vi "muPathSamplingFPGA2.vi"() -> ()   [LabVIEW 2017]
uses:
  <vilib>/rvi/Emulation/niFpgaSctlEmulationGetInTimedLoop.vi
  <vilib>/rvi/Emulation/niFpgaProcessEmulError.vi
  <vilib>/rvi/Emulation/niFpgaGetClockAttributes.vi
  <vilib>/rvi/Emulation/niFpgaEmulationReportErrorSimple.vi
  <vilib>/rvi/eio/common/nirviEmuTemplateMethod_errors.vi
  <vilib>/rvi/Emulation/niFpgaCriticalErrorInLSC.vi
  <vilib>/rvi/interface/RandomDataEmulation/niFpgaRandomDataHandleErrors.vi
  <vilib>/eio/EIONode/EIONode.xnode
  <vilib>/rvi/DataTransferAndStorage/Container/XNode/niFpgaContainer.xnode
  <vilib>/rvi/interface/RandomDataEmulation/nirviRandomDataFpgaReadWriteTemplate.vi
panel:
  out "samples":T1
  in  "Sampling Clock (uSec)":fxp<+/-,64,29>
  out "signalToInitialStageStop":bool
  out "y_pos_initial":fxp<+,16,16>
  out "x_pos_initial":fxp<+,16,16>
  out "ToRead":u32
  in  "Stage Clock (uSec)":fxp<+/-,64,29>
  in  "SettleCheckBuffer":u16
  out "b samples":fxp<+/-,64,32>[](array[numeric])
  out "a samples":fxp<+/-,64,32>[](array[numeric])
  out "y_FinalPos":fxp<+,16,16>
  out "x_FinalPos":fxp<+,16,16>
  out "direction":u16
  out "length":fxp<+,16,16>
  in  "deflection threshold":fxp<+/-,20,5>
  in  "z threshold":fxp<+/-,20,5>
  in  "y threshold":fxp<+/-,20,5>
  in  "x threshold":fxp<+/-,20,5>
  in  "stageIndicator":u8
  in  "z control":T2
  out "zControlMode":bool
  in  "Z Clock (uSec)":fxp<+/-,64,29>
  in  "deflection control":T2
  out "z output":fxp<+/-,64,29>
  out "deflection sensor":fxp<+/-,20,5>
  in  "XY Clock (uSec)":fxp<+/-,64,29>
  out "y_pos":fxp<+,16,16>
  out "x_pos":fxp<+,16,16>
  out "signalToStop":bool
  in  "x control":T2
  out "x output":fxp<+/-,64,29>
  out "x sensor":fxp<+/-,20,5>
  in  "y control":T2
  out "y output":fxp<+/-,64,29>
  out "y sensor":fxp<+/-,20,5>
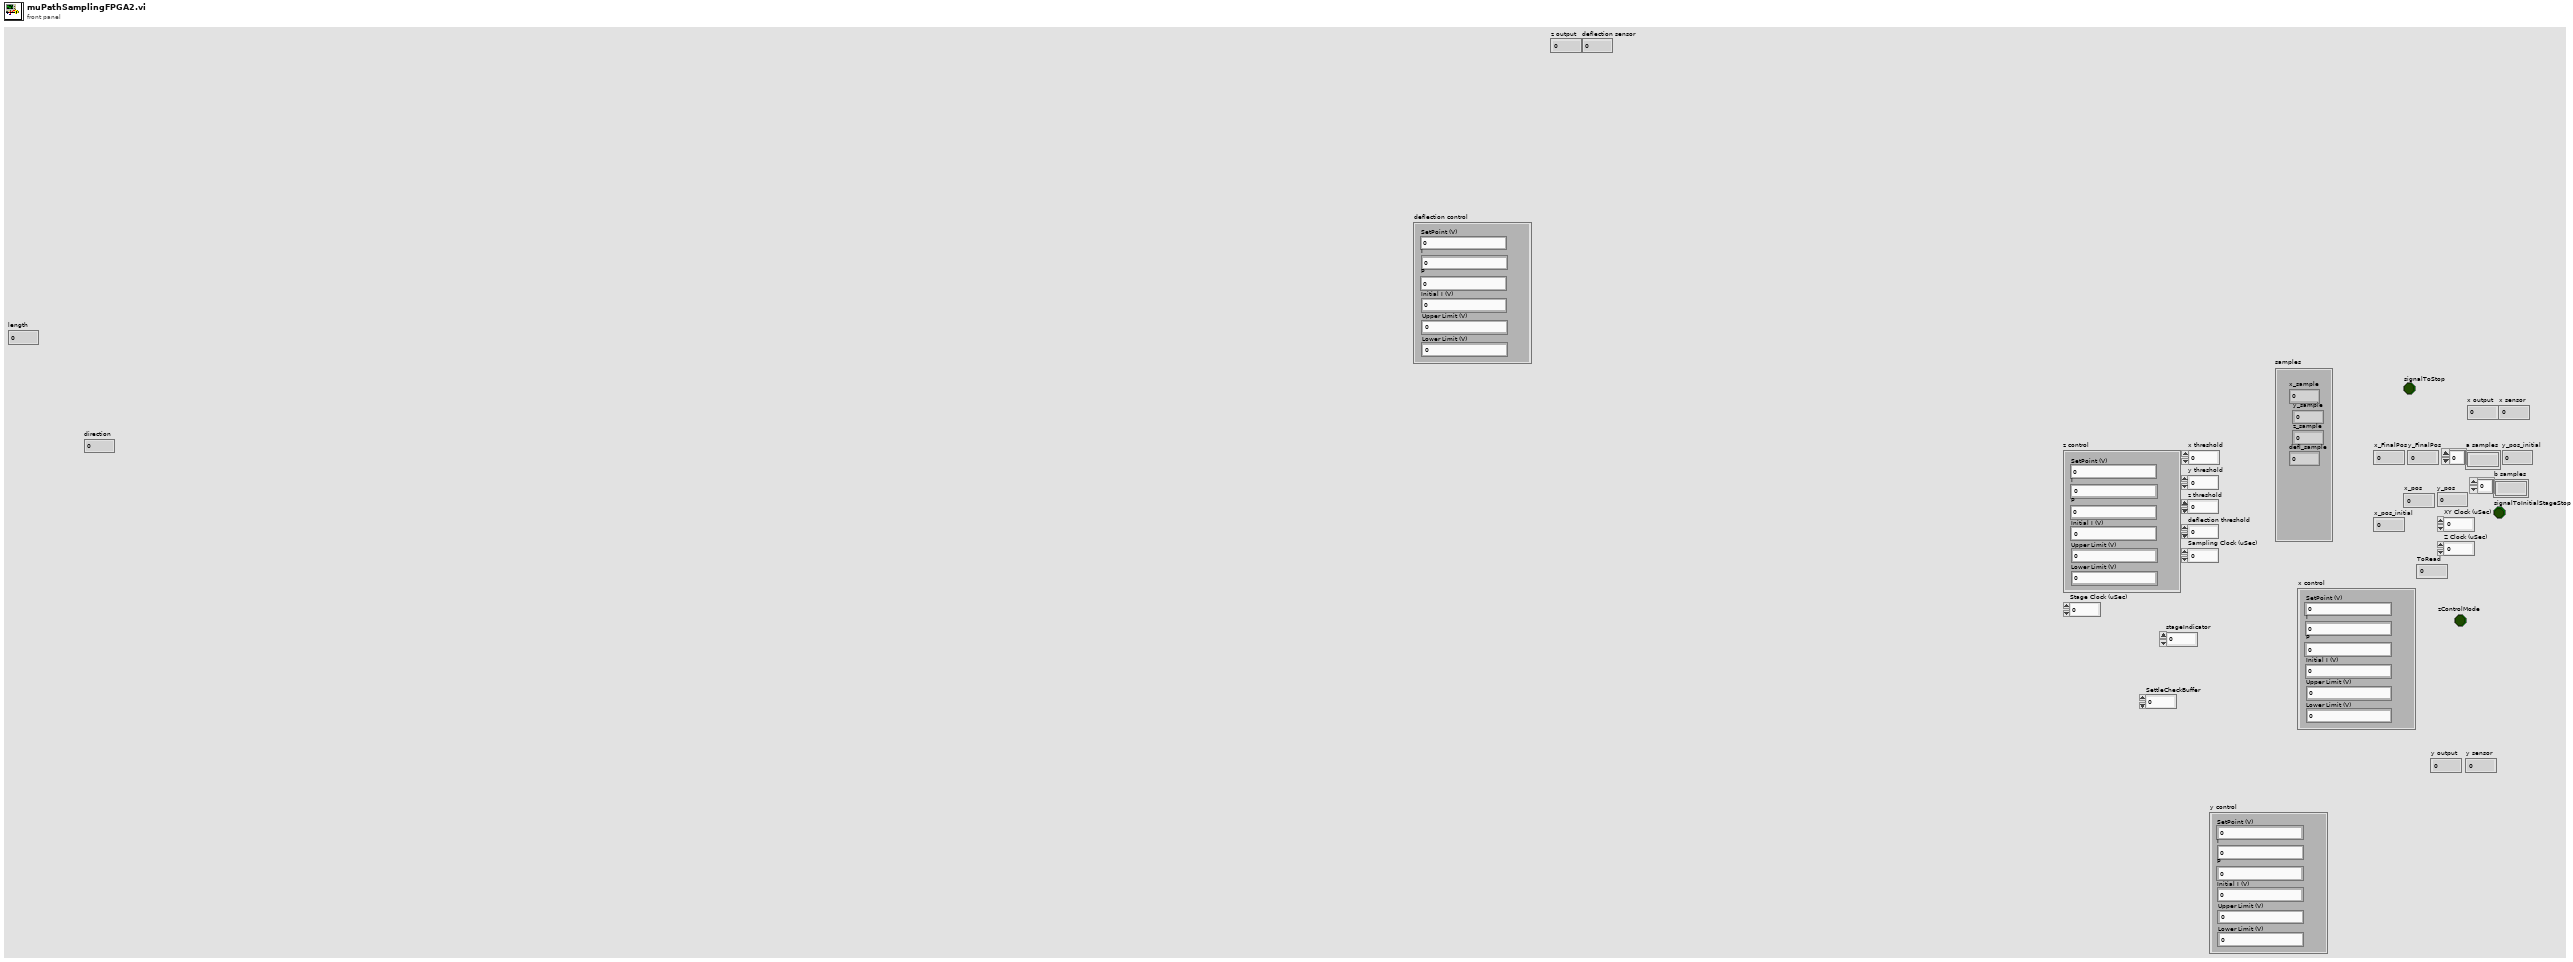
[diagram p1: front panel]
types:
  T1 = cluster{"y_sample":fxp<+/-,30,5>, "x_sample":fxp<+/-,30,5>, "z_sample":fxp<+/-,30,5>, "defl_sample":fxp<+/-,30,5>}
  T2 = cluster{"SetPoint (V)":fxp<+/-,20,5>, "I":fxp<+/-,20,5>, "P":fxp<+/-,20,5>, "Initial I (V)":fxp<+/-,64,29>, "Upper Limit (V)":fxp<+/-,64,29>, "Lower Limit (V)":fxp<+/-,64,29>}
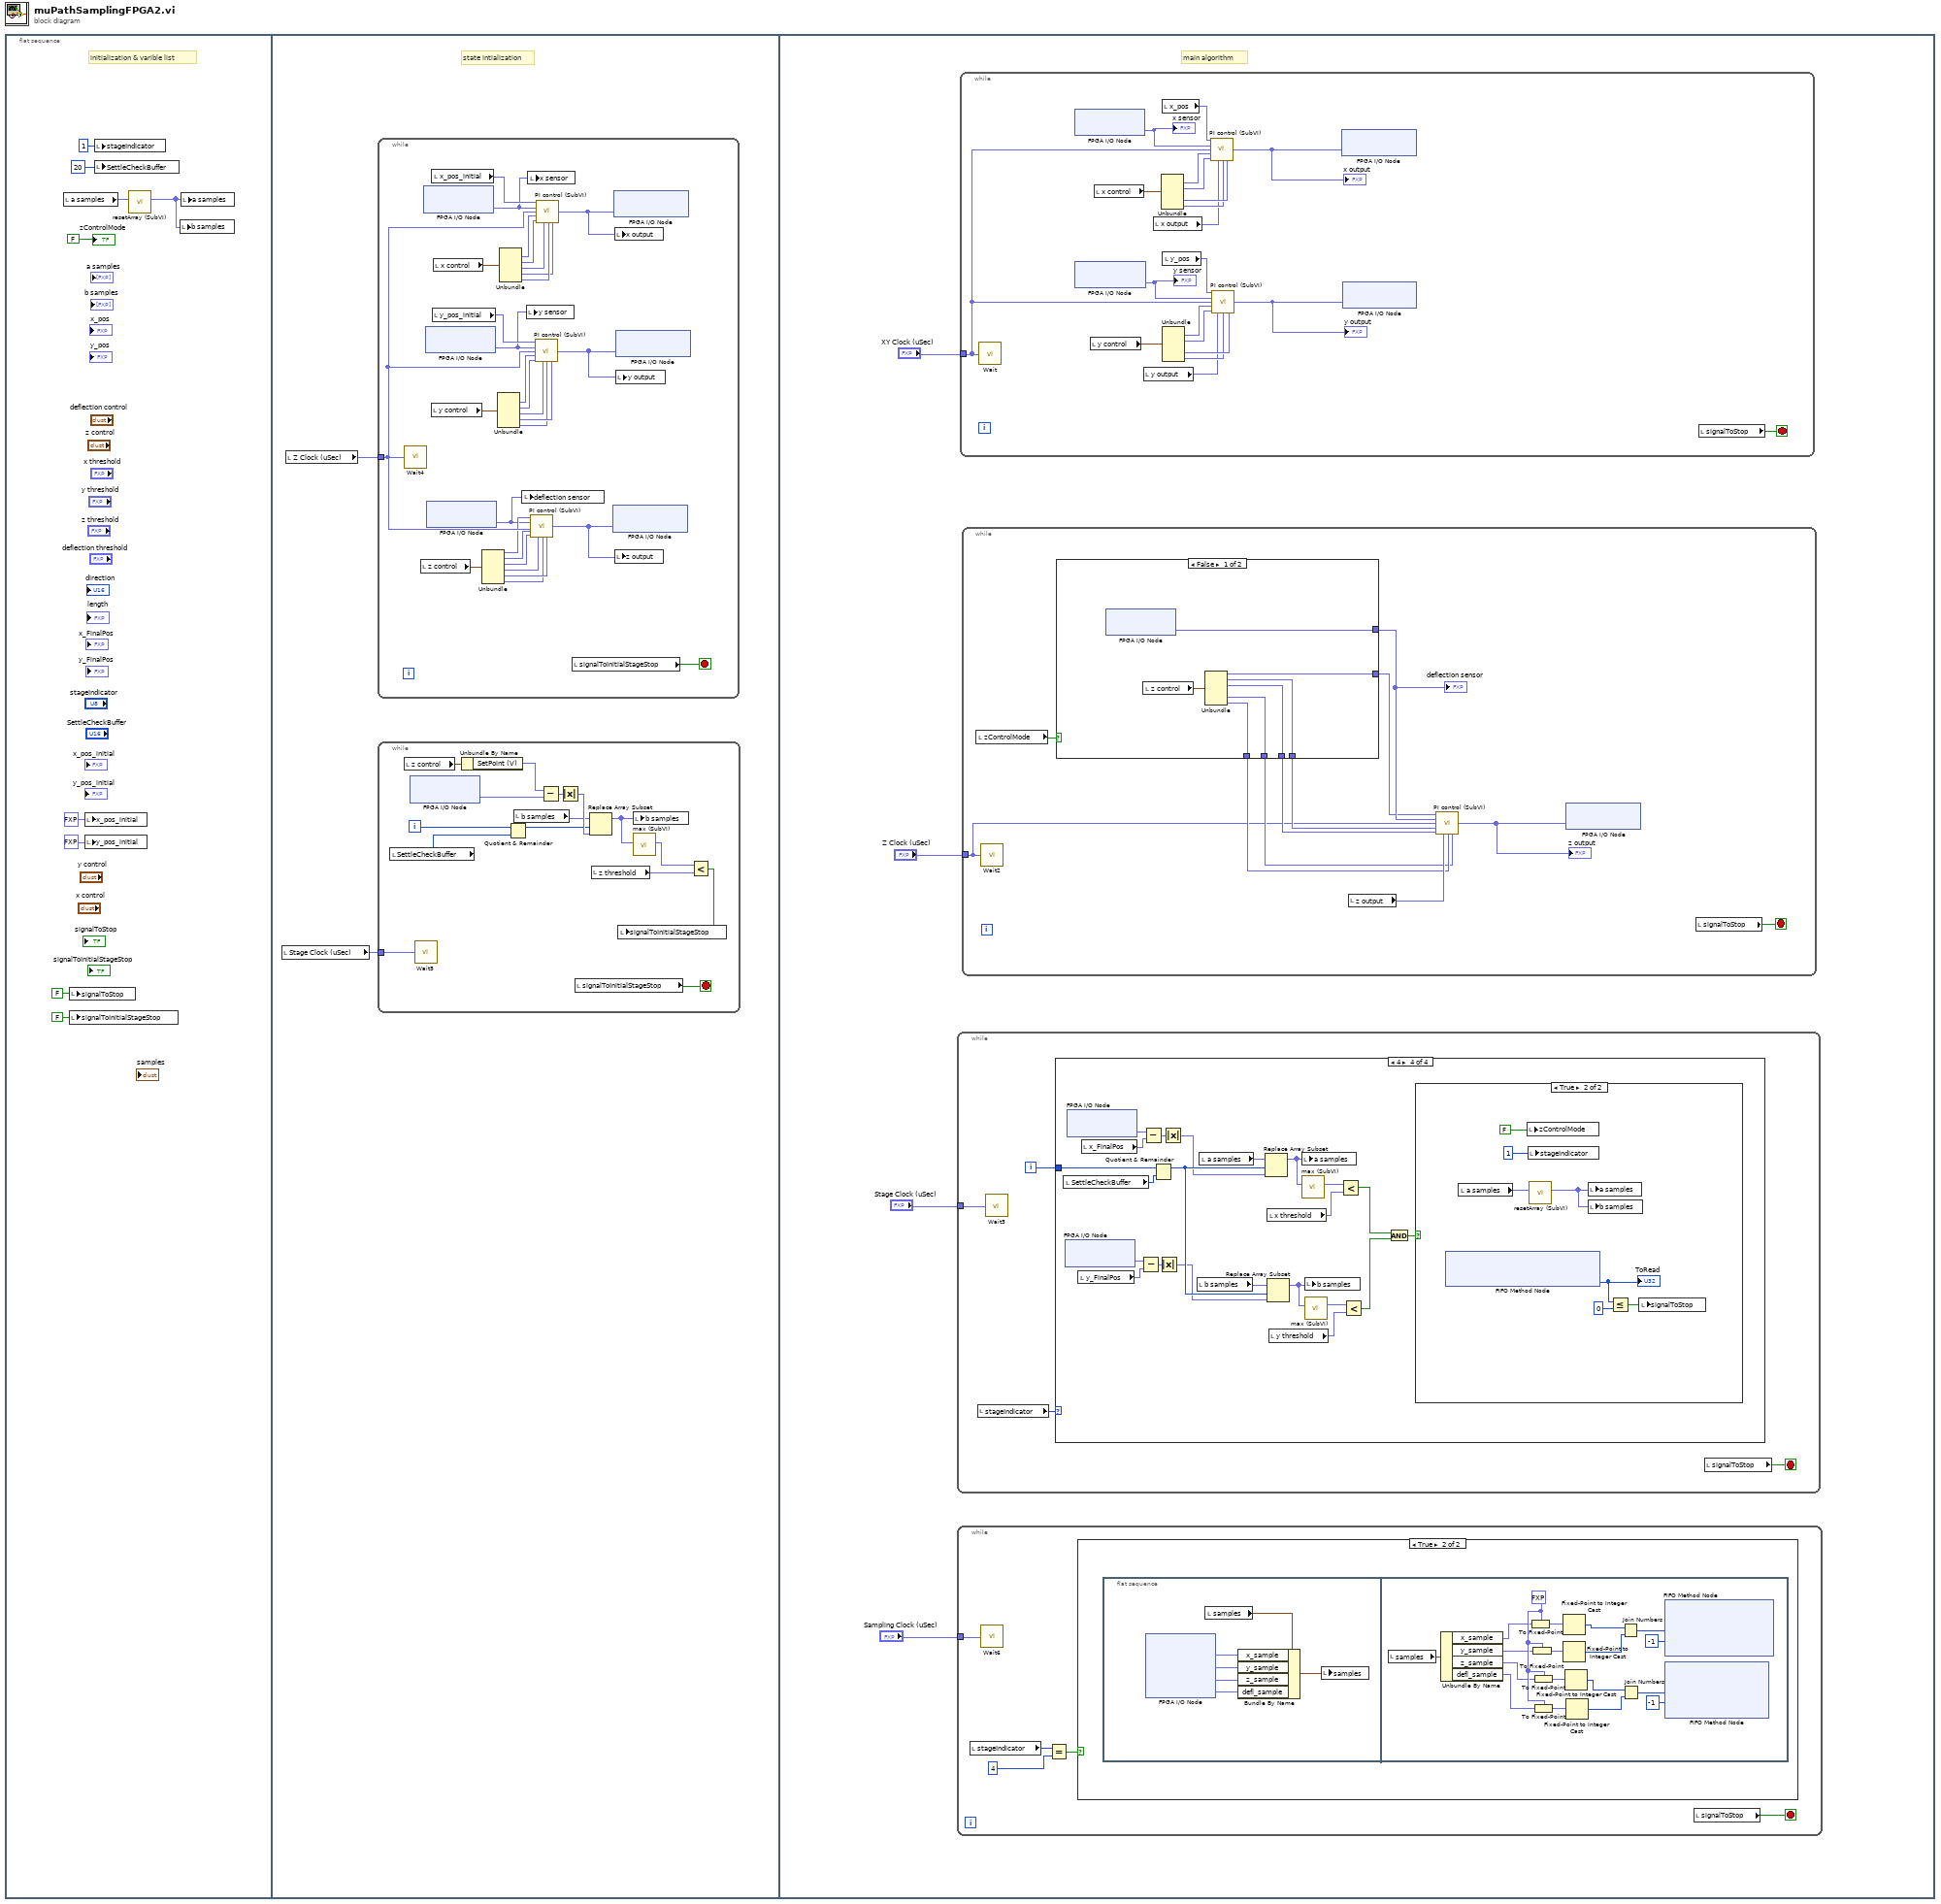
[diagram p0: block diagram]
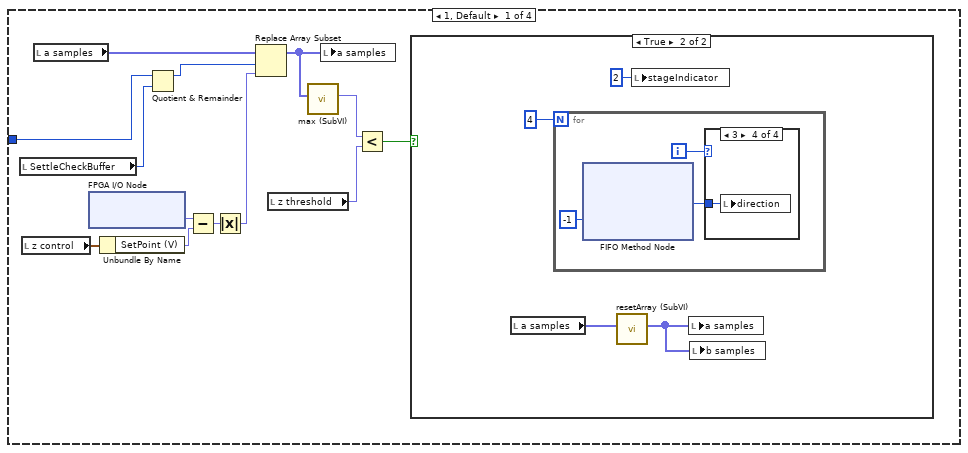
[diagram p3: hidden frame]
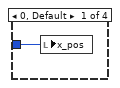
[diagram p5: hidden frame]
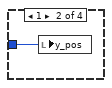
[diagram p6: hidden frame]
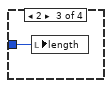
[diagram p7: hidden frame]
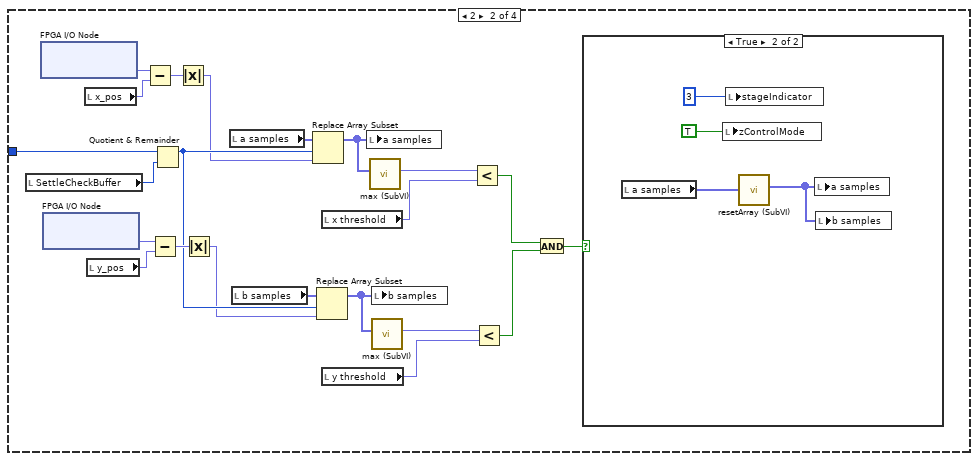
[diagram p8: hidden frame]
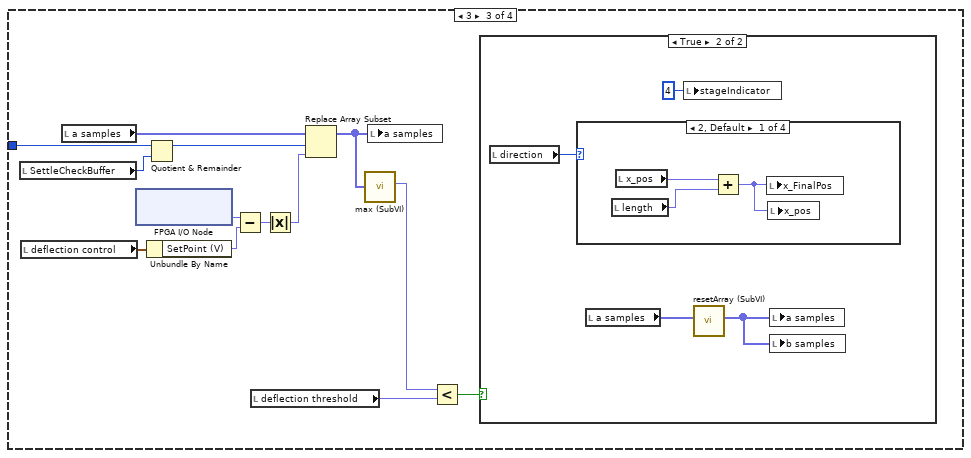
[diagram p10: hidden frame]
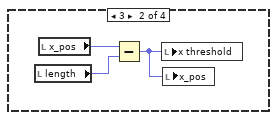
[diagram p12: hidden frame]
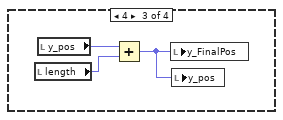
[diagram p13: hidden frame]
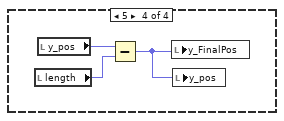
[diagram p14: hidden frame]
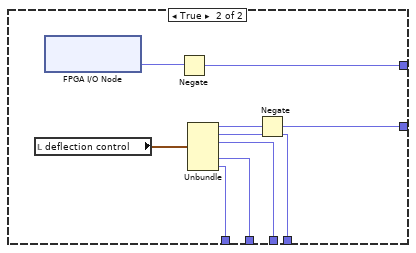
[diagram p16: hidden frame]
diagram:
  n1 = flat-sequence {
    frame #0 {
      # "initialization & varible list"
      n2 = local read "a samples"() -> (w6:fxp<+/-,64,32>[])
      n3 = local write "signalToStop"(FALSE ("signalToStop")) -> ()
      n4 = local write "signalToInitialStageStop"(FALSE ("signalToInitialStageStop")) -> ()
      n5 = local write "x_pos_initial"(fxp<+,16,16> 0.0 ("x_pos_initial")) -> ()
      n6 = local write "y_pos_initial"(fxp<+,16,16> 0.0 ("y_pos_initial")) -> ()
      n7 = local write "stageIndicator"(u8 1 ("stageIndicator")) -> ()
      n8 = local write "SettleCheckBuffer"(u16 20 ("SettleCheckLen")) -> ()
      n9 = call "resetArray (SubVI).vi"("a samples in"=w6) -> ("a samples out"=w7:fxp<+/-,64,32>[])  [unwired: 10 in]
      n10 = local write "b samples"(w7) -> ()
      n11 = local write "a samples"(w7) -> ()
      "zControlMode" <- FALSE ("zControlMode")
    }
    frame #1 {
      # "state intialization"
      n12 = local read "Stage Clock (uSec)"() -> (w10:fxp<+/-,64,29>)
      n13 = local read "Z Clock (uSec)"() -> (w11:fxp<+/-,64,29>)
      n14 = while {
        tunnel: w11 -> [w30]
        stop <- w27 stop-if-true
        n15 = call "Wait4"("Count(uSec)"=w30) -> ()  [unwired: 1 out]
        n16 = local read "z control"() -> (w37:T2)
        n17 = xnode "FPGA I/O Node"() -> ("Mod1/AI0"=w47:fxp<+/-,20,5>)  [unwired: 1 in, 1 out]
        n18 = xnode "FPGA I/O Node"() -> ("Mod1/AI1"=w39:fxp<+/-,20,5>)  [unwired: 1 in, 1 out]
        n19 = xnode "FPGA I/O Node"() -> ("Mod1/AI2"=w28:fxp<+/-,20,5>)  [unwired: 1 in, 1 out]
        n20 = local read "y control"() -> (w46:T2)
        n21 = local read "x_pos_initial"() -> (w55:fxp<+,16,16>)
        n22 = local read "y_pos_initial"() -> (w40:fxp<+,16,16>)
        n23 = local read "x control"() -> (w54:T2)
        n24 = Unbundle(w37) -> ("SetPoint (V)"=w29:fxp<+/-,20,5>, "I"=w36:fxp<+/-,20,5>, "P"=w35:fxp<+/-,20,5>, "Initial I (V)"=w34:fxp<+/-,64,29>, "Upper Limit (V)"=w33:fxp<+/-,64,29>, "Lower Limit (V)"=w32:fxp<+/-,64,29>)
        n25 = Unbundle(w46) -> ("I"=w45:fxp<+/-,20,5>, "P"=w44:fxp<+/-,20,5>, "Initial I (V)"=w41:fxp<+/-,64,29>, "Upper Limit (V)"=w43:fxp<+/-,64,29>, "Lower Limit (V)"=w42:fxp<+/-,64,29>)  [unwired: 1 out]
        n26 = Unbundle(w54) -> ("I"=w53:fxp<+/-,20,5>, "P"=w52:fxp<+/-,20,5>, "Initial I (V)"=w51:fxp<+/-,64,29>, "Upper Limit (V)"=w49:fxp<+/-,64,29>, "Lower Limit (V)"=w50:fxp<+/-,64,29>)  [unwired: 1 out]
        n27 = local write "deflection sensor"(w28) -> ()
        n28 = local write "y sensor"(w39) -> ()
        n29 = local write "x sensor"(w47) -> ()
        n30 = call "PI control (SubVI).vi"("SetPoint"=w29, "Feedback"=w28, "Clock"=w30, "I"=w36, "P"=w35, "Initial I"=w34, "Lower Limit"=w32, "Upper Limit in"=w33) -> ("Output"=w31:fxp<+/-,64,29>)  [unwired: 7 in]
        n31 = call "PI control (SubVI).vi"("SetPoint"=w40, "Feedback"=w39, "Clock"=w30, "I"=w45, "P"=w44, "Initial I"=w41, "Lower Limit"=w42, "Upper Limit in"=w43) -> ("Output"=w38:fxp<+/-,64,29>)  [unwired: 7 in]
        n32 = call "PI control (SubVI).vi"("SetPoint"=w55, "Feedback"=w47, "Clock"=w30, "I"=w53, "P"=w52, "Initial I"=w51, "Lower Limit"=w50, "Upper Limit in"=w49) -> ("Output"=w48:fxp<+/-,64,29>)  [unwired: 7 in]
        n33 = local read "signalToInitialStageStop"() -> (w27:bool)
        n34 = xnode "FPGA I/O Node"("Mod8/AO2"=w31) -> ()  [unwired: 1 in, 1 out]
        n35 = xnode "FPGA I/O Node"("Mod8/AO0"=w48) -> ()  [unwired: 1 in, 1 out]
        n36 = local write "x output"(w48) -> ()
        n37 = local write "z output"(w31) -> ()
        n38 = xnode "FPGA I/O Node"("Mod8/AO1"=w38) -> ()  [unwired: 1 in, 1 out]
        n39 = local write "y output"(w38) -> ()
      }
      n40 = while {
        tunnel: w10 -> [w18]
        i -> [w17]
        stop <- w16 stop-if-true
        n41 = local read "SettleCheckBuffer"() -> (w19:u16)
        n42 = local read "z control"() -> (w14:T2)
        n43 = xnode "FPGA I/O Node"() -> ("Mod1/AI2"=w15:fxp<+/-,20,5>)  [unwired: 1 in, 1 out]
        n44 = call "Wait5"("Count(uSec)"=w18) -> ()  [unwired: 1 out]
        n45 = Unbundle By Name(w14) -> ("SetPoint (V)"=w13:fxp<+/-,20,5>)
        n46 = Quotient & Remainder(x=w17, y=w19) -> (x-y*floor(x/y)=w22:i32)  [unwired: 1 out]
        n47 = local read "b samples"() -> (w21:fxp<+/-,64,32>[])
        n48 = Subtract(x=w13, y=w15) -> (x-y=w20:fxp<+/-,21,6>)
        n49 = Absolute Value(x=w20) -> (abs(x)=w23:fxp<+,20,5>)
        n50 = local read "signalToInitialStageStop"() -> (w16:bool)
        n51 = Replace Array Subset(array=w21, new element=w23, index=w22) -> (w25:fxp<+/-,64,32>[])
        n52 = local read "z threshold"() -> (w26:fxp<+/-,20,5>)
        n53 = local write "b samples"(w25) -> ()
        n54 = call "max (SubVI).vi"("initialized array"=w25) -> ("y"=w24:fxp<+/-,64,32>)  [unwired: 10 in]
        n55 = Less?(x=w24, y=w26) -> (x < y?=w12:bool)
        n56 = local write "signalToInitialStageStop"(w12) -> ()
      }
    }
    frame #2 {
      # "main algorithm"
      n57 = while {
        tunnel: "Stage Clock (uSec)" -> [w90]
        i -> [w89]
        stop <- w92 stop-if-true
        n58 = local read "stageIndicator"() -> (w91:u8)
        n59 = call "Wait3"("Count(uSec)"=w90) -> ()  [unwired: 1 out]
        n60 = case shown="4" w91 {
          tunnel: w89 -> [w104 w131 w151 w186]
          frame 1, Default {
            n61 = local read "SettleCheckBuffer"() -> (w103:u16)
            n62 = local read "z control"() -> (w99:T2)
            n63 = local read "a samples"() -> (w102:fxp<+/-,64,32>[])
            n64 = xnode "FPGA I/O Node"() -> ("Mod1/AI2"=w100:fxp<+/-,20,5>)  [unwired: 1 in, 1 out]
            n65 = Unbundle By Name(w99) -> ("SetPoint (V)"=w98:fxp<+/-,20,5>)
            n66 = Quotient & Remainder(x=w104, y=w103) -> (x-y*floor(x/y)=w97:i32)  [unwired: 1 out]
            n67 = Subtract(x=w100, y=w98) -> (x-y=w101:fxp<+/-,21,6>)
            n68 = Absolute Value(x=w101) -> (abs(x)=w96:fxp<+,20,5>)
            n69 = Replace Array Subset(array=w102, new element=w96, index=w97) -> (w94:fxp<+/-,64,32>[])
            n70 = local read "z threshold"() -> (w95:fxp<+/-,20,5>)
            n71 = call "max (SubVI).vi"("initialized array"=w94) -> ("y"=w93:fxp<+/-,64,32>)  [unwired: 10 in]
            n72 = local write "a samples"(w94) -> ()
            n73 = Less?(x=w93, y=w95) -> (x < y?=w105:bool)
            n74 = case shown="True" w105 {
              frame False {
              }
              frame True {
                n75 = local read "a samples"() -> (w107:fxp<+/-,64,32>[])
                n76 = for {
                  N: 4 -> [_]
                  i -> [w112]
                  n77 = xnode ("FIFO Method Node")("Timeout"=-1) -> ("Element"=w110:u16)  [unwired: 1 in, 2 out]
                  n78 = case shown="3" w112 {
                    tunnel: w110 -> [w113 w114 w115 w116]
                    frame 0, Default {
                      n79 = local write "x_pos"(w113) -> ()
                    }
                    frame 1 {
                      n80 = local write "y_pos"(w114) -> ()
                    }
                    frame 2 {
                      n81 = local write "length"(w115) -> ()
                    }
                    frame 3 {
                      n82 = local write "direction"(w116) -> ()
                    }
                  }
                }
                n83 = call "resetArray (SubVI).vi"("a samples in"=w107) -> ("a samples out"=w106:fxp<+/-,64,32>[])  [unwired: 10 in]
                n84 = local write "stageIndicator"(u8 2 ("stageIndicator")) -> ()
                n85 = local write "a samples"(w106) -> ()
                n86 = local write "b samples"(w106) -> ()
              }
            }
          }
          frame 2 {
            n87 = local read "SettleCheckBuffer"() -> (w130:u16)
            n88 = xnode "FPGA I/O Node"() -> ("Mod1/AI0"=w137:fxp<+/-,20,5>)  [unwired: 1 in, 1 out]
            n89 = xnode "FPGA I/O Node"() -> ("Mod1/AI1"=w135:fxp<+/-,20,5>)  [unwired: 1 in, 1 out]
            n90 = local read "x_pos"() -> (w134:fxp<+,16,16>)
            n91 = local read "y_pos"() -> (w133:fxp<+,16,16>)
            n92 = Subtract(x=w137, y=w134) -> (x-y=w138:fxp<+/-,33,18>)
            n93 = Subtract(x=w135, y=w133) -> (x-y=w136:fxp<+/-,33,18>)
            n94 = Quotient & Remainder(x=w131, y=w130) -> (x-y*floor(x/y)=w128:i32)  [unwired: 1 out]
            n95 = Absolute Value(x=w138) -> (abs(x)=w126:fxp<+,32,17>)
            n96 = Absolute Value(x=w136) -> (abs(x)=w125:fxp<+,32,17>)
            n97 = local read "a samples"() -> (w129:fxp<+/-,64,32>[])
            n98 = local read "b samples"() -> (w127:fxp<+/-,64,32>[])
            n99 = Replace Array Subset(array=w129, new element=w126, index=w128) -> (w119:fxp<+/-,64,32>[])
            n100 = Replace Array Subset(array=w127, new element=w125, index=w128) -> (w117:fxp<+/-,64,32>[])
            n101 = local read "x threshold"() -> (w124:fxp<+/-,20,5>)
            n102 = local read "y threshold"() -> (w123:fxp<+/-,20,5>)
            n103 = local write "a samples"(w119) -> ()
            n104 = call "max (SubVI).vi"("initialized array"=w119) -> ("y"=w120:fxp<+/-,64,32>)  [unwired: 10 in]
            n105 = local write "b samples"(w117) -> ()
            n106 = call "max (SubVI).vi"("initialized array"=w117) -> ("y"=w118:fxp<+/-,64,32>)  [unwired: 10 in]
            n107 = Less?(x=w120, y=w124) -> (x < y?=w122:bool)
            n108 = Less?(x=w118, y=w123) -> (x < y?=w121:bool)
            n109 = And(x=w122, y=w121) -> (x .and. y?=w132:bool)
            n110 = case shown="True" w132 {
              frame False {
              }
              frame True {
                n111 = local read "a samples"() -> (w140:fxp<+/-,64,32>[])
                n112 = local write "zControlMode"(TRUE ("signalToStop")) -> ()
                n113 = local write "stageIndicator"(u8 3 ("stageIndicator")) -> ()
                n114 = call "resetArray (SubVI).vi"("a samples in"=w140) -> ("a samples out"=w139:fxp<+/-,64,32>[])  [unwired: 10 in]
                n115 = local write "a samples"(w139) -> ()
                n116 = local write "b samples"(w139) -> ()
              }
            }
          }
          frame 3 {
            n117 = local read "SettleCheckBuffer"() -> (w150:u16)
            n118 = local read "deflection control"() -> (w153:T2)
            n119 = local read "a samples"() -> (w148:fxp<+/-,64,32>[])
            n120 = xnode "FPGA I/O Node"() -> ("Mod1/AI3"=w154:fxp<+/-,20,5>)  [unwired: 1 in, 1 out]
            n121 = Quotient & Remainder(x=w151, y=w150) -> (x-y*floor(x/y)=w149:i32)  [unwired: 1 out]
            n122 = Unbundle By Name(w153) -> ("SetPoint (V)"=w152:fxp<+/-,20,5>)
            n123 = Subtract(x=w154, y=w152) -> (x-y=w155:fxp<+/-,21,6>)
            n124 = local read "deflection threshold"() -> (w145:fxp<+/-,20,5>)
            n125 = Absolute Value(x=w155) -> (abs(x)=w147:fxp<+,20,5>)
            n126 = Replace Array Subset(array=w148, new element=w147, index=w149) -> (w144:fxp<+/-,64,32>[])
            n127 = call "max (SubVI).vi"("initialized array"=w144) -> ("y"=w143:fxp<+/-,64,32>)  [unwired: 10 in]
            n128 = local write "a samples"(w144) -> ()
            n129 = Less?(x=w143, y=w145) -> (x < y?=w146:bool)
            n130 = case shown="True" w146 {
              frame False {
              }
              frame True {
                n131 = local read "direction"() -> (w158:u16)
                n132 = case shown="2, Default" w158 {
                  frame 2, Default {
                    n133 = local read "length"() -> (w161:fxp<+,16,16>)
                    n134 = local read "x_pos"() -> (w162:fxp<+,16,16>)
                    n135 = Add(x=w162, y=w161) -> (x+y=w160:fxp<+,17,17>)
                    n136 = local write "x_FinalPos"(w160) -> ()
                    n137 = local write "x_pos"(w160) -> ()
                  }
                  frame 3 {
                    n138 = local read "length"() -> (w164:fxp<+,16,16>)
                    n139 = local read "x_pos"() -> (w165:fxp<+,16,16>)
                    n140 = Subtract(x=w165, y=w164) -> (x-y=w163:fxp<+/-,17,17>)
                    n141 = local write "x threshold"(w163) -> ()
                    n142 = local write "x_pos"(w163) -> ()
                  }
                  frame 4 {
                    n143 = local read "length"() -> (w167:fxp<+,16,16>)
                    n144 = local read "y_pos"() -> (w168:fxp<+,16,16>)
                    n145 = Add(x=w168, y=w167) -> (x+y=w166:fxp<+,17,17>)
                    n146 = local write "y_FinalPos"(w166) -> ()
                    n147 = local write "y_pos"(w166) -> ()
                  }
                  frame 5 {
                    n148 = local read "length"() -> (w170:fxp<+,16,16>)
                    n149 = local read "y_pos"() -> (w171:fxp<+,16,16>)
                    n150 = Subtract(x=w171, y=w170) -> (x-y=w169:fxp<+/-,17,17>)
                    n151 = local write "y_FinalPos"(w169) -> ()
                    n152 = local write "y_pos"(w169) -> ()
                  }
                }
                n153 = local read "a samples"() -> (w156:fxp<+/-,64,32>[])
                n154 = local write "stageIndicator"(u8 4 ("stageIndicator")) -> ()
                n155 = call "resetArray (SubVI).vi"("a samples in"=w156) -> ("a samples out"=w157:fxp<+/-,64,32>[])  [unwired: 10 in]
                n156 = local write "a samples"(w157) -> ()
                n157 = local write "b samples"(w157) -> ()
              }
            }
          }
          frame 4 {
            n158 = local read "SettleCheckBuffer"() -> (w185:u16)
            n159 = xnode "FPGA I/O Node"() -> ("Mod1/AI1"=w191:fxp<+/-,20,5>)  [unwired: 1 in, 1 out]
            n160 = xnode "FPGA I/O Node"() -> ("Mod1/AI0"=w193:fxp<+/-,20,5>)  [unwired: 1 in, 1 out]
            n161 = local read "y_FinalPos"() -> (w187:fxp<+,16,16>)
            n162 = local read "x_FinalPos"() -> (w188:fxp<+,16,16>)
            n163 = Subtract(x=w191, y=w187) -> (x-y=w190:fxp<+/-,33,18>)
            n164 = Subtract(x=w193, y=w188) -> (x-y=w192:fxp<+/-,33,18>)
            n165 = Quotient & Remainder(x=w186, y=w185) -> (x-y*floor(x/y)=w184:i32)  [unwired: 1 out]
            n166 = Absolute Value(x=w190) -> (abs(x)=w183:fxp<+,32,17>)
            n167 = Absolute Value(x=w192) -> (abs(x)=w182:fxp<+,32,17>)
            n168 = local read "b samples"() -> (w180:fxp<+/-,64,32>[])
            n169 = local read "a samples"() -> (w181:fxp<+/-,64,32>[])
            n170 = Replace Array Subset(array=w181, new element=w182, index=w184) -> (w172:fxp<+/-,64,32>[])
            n171 = Replace Array Subset(array=w180, new element=w183, index=w184) -> (w175:fxp<+/-,64,32>[])
            n172 = local read "x threshold"() -> (w179:fxp<+/-,20,5>)
            n173 = local read "y threshold"() -> (w178:fxp<+/-,20,5>)
            n174 = local write "a samples"(w172) -> ()
            n175 = call "max (SubVI).vi"("initialized array"=w172) -> ("y"=w173:fxp<+/-,64,32>)  [unwired: 10 in]
            n176 = local write "b samples"(w175) -> ()
            n177 = call "max (SubVI).vi"("initialized array"=w175) -> ("y"=w174:fxp<+/-,64,32>)  [unwired: 10 in]
            n178 = Less?(x=w173, y=w179) -> (x < y?=w177:bool)
            n179 = Less?(x=w174, y=w178) -> (x < y?=w176:bool)
            n180 = And(x=w177, y=w176) -> (x .and. y?=w189:bool)
            n181 = case shown="True" w189 {
              frame False {
              }
              frame True {
                n182 = xnode ("FIFO Method Node")() -> ("Number of Elements to Read"=w198:u32)  [unwired: 1 in, 1 out]
                "ToRead" <- w198
                n183 = local read "a samples"() -> (w195:fxp<+/-,64,32>[])
                n184 = local write "zControlMode"(FALSE ("zControlMode")) -> ()
                n185 = local write "stageIndicator"(u8 1 ("stageIndicator")) -> ()
                n186 = call "resetArray (SubVI).vi"("a samples in"=w195) -> ("a samples out"=w194:fxp<+/-,64,32>[])  [unwired: 10 in]
                n187 = local write "a samples"(w194) -> ()
                n188 = local write "b samples"(w194) -> ()
                n189 = Less Or Equal?(x=w198, y=u32 0) -> (x <= y?=w196:bool)
                n190 = local write "signalToStop"(w196) -> ()
              }
            }
          }
        }
        n191 = local read "signalToStop"() -> (w92:bool)
      }
      n192 = while {
        tunnel: "Sampling Clock (uSec)" -> [w64]
        stop <- w63 stop-if-true
        n193 = local read "stageIndicator"() -> (w62:u8)
        n194 = call "Wait6"("Count(uSec)"=w64) -> ()  [unwired: 1 out]
        n195 = Equal?(x=w62, y=u8 4) -> (x = y?=w60:bool)
        n196 = case shown="True" w60 {
          frame False {
          }
          frame True {
            n197 = flat-sequence {
              frame #0 {
                n198 = xnode "FPGA I/O Node"() -> ("Mod1/AI0"=w69:fxp<+/-,20,5>, "Mod1/AI1"=w68:fxp<+/-,20,5>, "Mod1/AI2"=w67:fxp<+/-,20,5>, "Mod1/AI3"=w66:fxp<+/-,20,5>)  [unwired: 4 in, 4 out]
                n199 = local read "samples"() -> (w70:T1)
                n200 = Bundle By Name(cluster=w70, "x_sample"=w69, "y_sample"=w68, "z_sample"=w67, "defl_sample"=w66) -> (w65:T1)
                n201 = local write "samples"(w65) -> ()
              }
              frame #1 {
                w88 = fxp<+/-,32,16> 0.0 ("fixed-point type")
                n202 = local read "samples"() -> (w75:T1)
                n203 = Unbundle By Name(w75) -> ("x_sample"=w71:fxp<+/-,30,5>, "y_sample"=w72:fxp<+/-,30,5>, "z_sample"=w73:fxp<+/-,30,5>, "defl_sample"=w74:fxp<+/-,30,5>)
                n204 = To Fixed-Point(fixed-point type=w88, number=w71) -> (fixed-point=w87:fxp<+/-,32,16>)
                n205 = To Fixed-Point(fixed-point type=w88, number=w72) -> (fixed-point=w86:fxp<+/-,32,16>)
                n206 = To Fixed-Point(fixed-point type=w88, number=w73) -> (fixed-point=w85:fxp<+/-,32,16>)
                n207 = To Fixed-Point(fixed-point type=w88, number=w74) -> (fixed-point=w84:fxp<+/-,32,16>)
                n208 = Fixed-Point to Integer Cast(1:w86) -> (0:w82:i32)
                n209 = Fixed-Point to Integer Cast(1:w87) -> (0:w83:i32)
                n210 = Fixed-Point to Integer Cast(1:w85) -> (0:w81:i32)
                n211 = Fixed-Point to Integer Cast(1:w84) -> (0:w80:i32)
                n212 = Join Numbers(hi=w83, lo=w82) -> ((hi.lo)=w79:u64)
                n213 = Join Numbers(hi=w81, lo=w80) -> ((hi.lo)=w77:u64)
                n214 = xnode ("FIFO Method Node")("Element"=w79, "Timeout"=-1) -> ()  [unwired: 1 in, 2 out]
                n215 = xnode ("FIFO Method Node")("Element"=w77, "Timeout"=-1) -> ()  [unwired: 1 in, 2 out]
              }
            }
          }
        }
        n216 = local read "signalToStop"() -> (w63:bool)
      }
      n217 = while {
        tunnel: "XY Clock (uSec)" -> [w235]
        stop <- w232 stop-if-true
        n218 = call "Wait"("Count(uSec)"=w235) -> ()  [unwired: 1 out]
        n219 = xnode "FPGA I/O Node"() -> ("Mod1/AI0"=w241:fxp<+/-,20,5>)  [unwired: 1 in, 1 out]
        "x sensor" <- w241
        n220 = xnode "FPGA I/O Node"() -> ("Mod1/AI1"=w247:fxp<+/-,20,5>)  [unwired: 1 in, 1 out]
        "y sensor" <- w247
        n221 = local read "y control"() -> (w228:T2)
        n222 = local read "x control"() -> (w229:T2)
        n223 = local read "y output"() -> (w230:fxp<+/-,64,29>)
        n224 = local read "x output"() -> (w231:fxp<+/-,64,29>)
        n225 = Unbundle(w229) -> ("I"=w236:fxp<+/-,20,5>, "P"=w237:fxp<+/-,20,5>, "Upper Limit (V)"=w239:fxp<+/-,64,29>, "Lower Limit (V)"=w238:fxp<+/-,64,29>)  [unwired: 2 out]
        n226 = local read "x_pos"() -> (w233:fxp<+,16,16>)
        n227 = local read "y_pos"() -> (w234:fxp<+,16,16>)
        n228 = Unbundle(w228) -> ("I"=w242:fxp<+/-,20,5>, "P"=w243:fxp<+/-,20,5>, "Upper Limit (V)"=w245:fxp<+/-,64,29>, "Lower Limit (V)"=w244:fxp<+/-,64,29>)  [unwired: 2 out]
        n229 = call "PI control (SubVI).vi"("SetPoint"=w233, "Feedback"=w241, "Clock"=w235, "I"=w236, "P"=w237, "Initial I"=w231, "Lower Limit"=w238, "Upper Limit in"=w239) -> ("Output"=w240:fxp<+/-,64,29>)  [unwired: 7 in]
        "x output" <- w240
        n230 = call "PI control (SubVI).vi"("SetPoint"=w234, "Feedback"=w247, "Clock"=w235, "I"=w242, "P"=w243, "Initial I"=w230, "Lower Limit"=w244, "Upper Limit in"=w245) -> ("Output"=w246:fxp<+/-,64,29>)  [unwired: 7 in]
        "y output" <- w246
        n231 = xnode "FPGA I/O Node"("Mod8/AO0"=w240) -> ()  [unwired: 1 in, 1 out]
        n232 = xnode "FPGA I/O Node"("Mod8/AO1"=w246) -> ()  [unwired: 1 in, 1 out]
        n233 = local read "signalToStop"() -> (w232:bool)
      }
      n234 = while {
        tunnel: "Z Clock (uSec)" -> [w201]
        stop <- w210 stop-if-true
        n235 = local read "zControlMode"() -> (w208:bool)
        n236 = call "Wait2"("Count(uSec)"=w201) -> ()  [unwired: 1 out]
        n237 = case shown="False" w208 {
          tunnel: [w217 w226] -> w207
          tunnel: [w216 w223] -> w206
          tunnel: [w212 w222] -> w205
          tunnel: [w213 w221] -> w204
          tunnel: [w215 w220] -> w203
          tunnel: [w214 w219] -> w202
          frame False {
            n238 = xnode "FPGA I/O Node"() -> ("Mod1/AI2"=w217:fxp<+/-,20,5>)  [unwired: 1 in, 1 out]
            n239 = local read "z control"() -> (w218:T2)
            n240 = Unbundle(w218) -> ("SetPoint (V)"=w216:fxp<+/-,20,5>, "I"=w212:fxp<+/-,20,5>, "P"=w213:fxp<+/-,20,5>, "Upper Limit (V)"=w214:fxp<+/-,64,29>, "Lower Limit (V)"=w215:fxp<+/-,64,29>)  [unwired: 1 out]
          }
          frame True {
            n241 = local read "deflection control"() -> (w225:T2)
            n242 = xnode "FPGA I/O Node"() -> ("Mod1/AI3"=w227:fxp<+/-,20,5>)  [unwired: 1 in, 1 out]
            n243 = Negate(x=w227) -> (-x=w226:fxp<+/-,21,6>)
            n244 = Unbundle(w225) -> ("SetPoint (V)"=w224:fxp<+/-,20,5>, "I"=w222:fxp<+/-,20,5>, "P"=w221:fxp<+/-,20,5>, "Upper Limit (V)"=w219:fxp<+/-,64,29>, "Lower Limit (V)"=w220:fxp<+/-,64,29>)  [unwired: 1 out]
            n245 = Negate(x=w224) -> (-x=w223:fxp<+/-,21,6>)
          }
        }
        "deflection sensor" <- w207
        n246 = local read "z output"() -> (w209:fxp<+/-,64,29>)
        n247 = call "PI control (SubVI).vi"("SetPoint"=w206, "Feedback"=w207, "Clock"=w201, "I"=w205, "P"=w204, "Initial I"=w209, "Lower Limit"=w203, "Upper Limit in"=w202) -> ("Output"=w211:fxp<+/-,64,29>)  [unwired: 7 in]
        "z output" <- w211
        n248 = xnode "FPGA I/O Node"("Mod8/AO2"=w211) -> ()  [unwired: 1 in, 1 out]
        n249 = local read "signalToStop"() -> (w210:bool)
      }
    }
  }
